vi "EditValue.vi"(8 "error in (no error)":errorcluster, 10 "Bounds":T1, 11 "U32 D Element.lvclass":refnum<class "Bool D Element.lvclass">) -> (0 "error out":errorcluster, 1 "Tabbed out?":bool, 2 "Value changed?":bool, 3 "U32 D Element.lvclass":refnum<class "Bool D Element.lvclass">)   [LabVIEW 2018, in "D Datagrid Library.lvlib" / "Bool D Element.lvclass"]
uses:
  Bool D Element.lvclass
  <vilib>/Utility/miscctls.llb/LVRectTypeDef.ctl
  Bool D Element.lvclass/Bool D Element.ctl
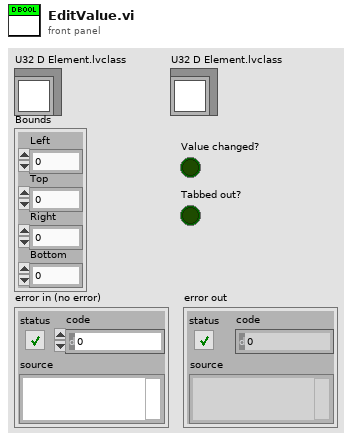
[diagram p1: front panel]
types:
  T1 = typedef "LVRectTypeDef.ctl" = cluster{"Left":i16, "Top":i16, "Right":i16, "Bottom":i16}
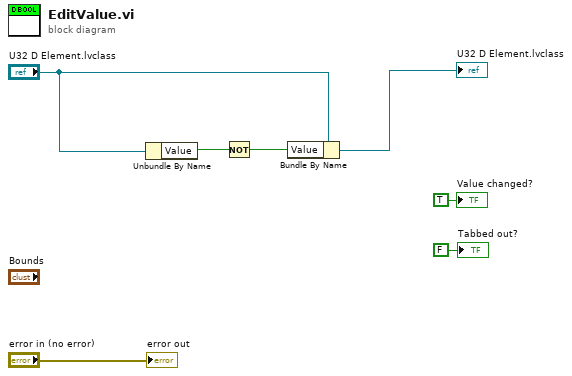
[diagram p0: block diagram]
diagram:
  n1 = Unbundle By Name("U32 D Element.lvclass") -> ("Value"=w3:bool)
  n2 = Not(x=w3) -> (.not. x?=w2:bool)
  n3 = Bundle By Name(cluster="U32 D Element.lvclass", "Value"=w2) -> (→"U32 D Element.lvclass":refnum<class "Bool D Element.lvclass">)
  "error out" <- "error in (no error)"
  "Value changed?" <- TRUE ("Generate newval event?")
  "Tabbed out?" <- FALSE ("Tabbed out?")
